vi "DEMO Lock.vi"(1 "Input":bool) -> (0 "Output":bool)   [LabVIEW 2012]
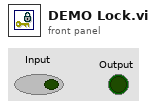
[diagram p1: front panel]
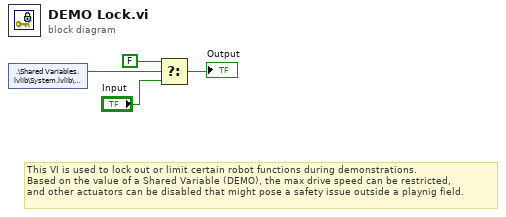
[diagram p0: block diagram]
diagram:
  # "This VI is used to lock out or limit certain robot functions during demonstrations.\nBased on the value of a Shared Variable (DEMO), the max drive speed can be restricted,\nand other actuators can be disabled that might pose a safety issue outside a playnig field."
  n1 = shared-variable ".\\Shared Variables.lvlib\\System.lvlib\\DEMO"() -> (w1:bool)  [unwired: 1 in, 1 out]
  n2 = Select(t=FALSE, s=w1, f="Input") -> (s? t:f=→"Output":bool)
